vi "Destructor.vi"(8 "error in":errorcluster, 11 "Michell Easydew in":refnum<class "Michell Easidew.lvclass">) -> (0 "error out":errorcluster, 3 "Michell Easydew out":refnum<class "Michell Easidew.lvclass">)   [LabVIEW 2011, in "Michell Easidew.lvclass"]
uses:
  Michell Easidew.lvclass
  Michell Easidew.lvclass/Michell Easidew.ctl
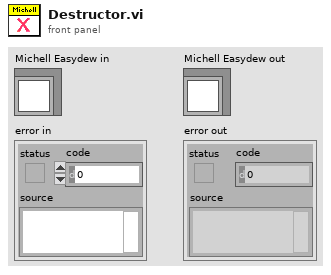
[diagram p1: front panel]
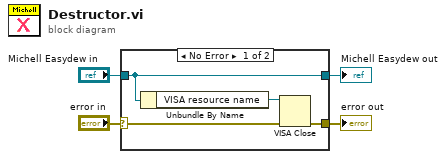
[diagram p0: block diagram]
diagram:
  n1 = case shown="No Error" "error in" {
    selector: "error in" -> [w6 w10]
    tunnel: [w5 w10] -> w3
    tunnel: [w8 w9] -> w1
    tunnel: "Michell Easydew in" -> [w8 w9]
    frame No Error {
      n2 = Unbundle By Name(w8) -> ("VISA resource name"=w7:refnum<visa-resource-name>)
      n3 = VISA Close(VISA resource name=w7, error in (no error)=w6) -> (error out=w5:errorcluster)
    }
    frame Error {
    }
  }
  "error out" <- w3
  "Michell Easydew out" <- w1
